vi "Illuminace (SubVI).vi"(5 "R Offset":dbl, 6 "Interval":dbl=1.0, 7 "IR Offset":dbl, 8 "Period (> 3s)":dbl=10.0, 9 "Width":i32, 10 "% Threshold":dbl, 11 "Filtered Signal":dynamicdata(waveform)) -> (0 "waveform out":waveform(dbl), 1 "Imax IR":dbl, 2 "Imin R":dbl, 3 "Imax R":dbl, 4 "Imin IR":dbl)   [LabVIEW 2021]
uses:
  <vilib>/Analysis/baseanly.llb/Mean (DBL).vi
  <vilib>/Waveform/WDTOps.llb/WDT Get Waveform Subset DBL.vi
  <vilib>/Analysis/NI_AAL_SigProc.lvlib
  <vilib>/Analysis/NI_AALBase.lvlib
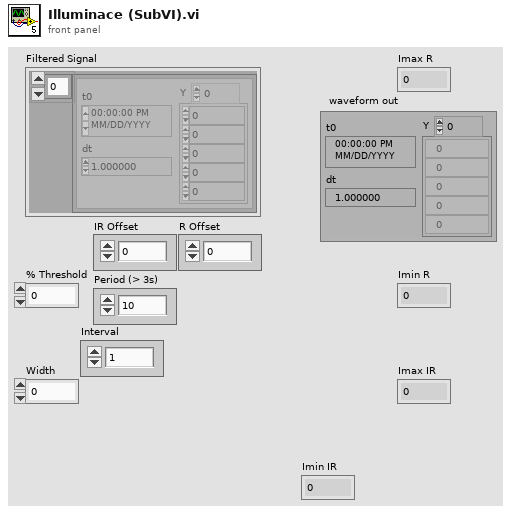
[diagram p1: front panel]
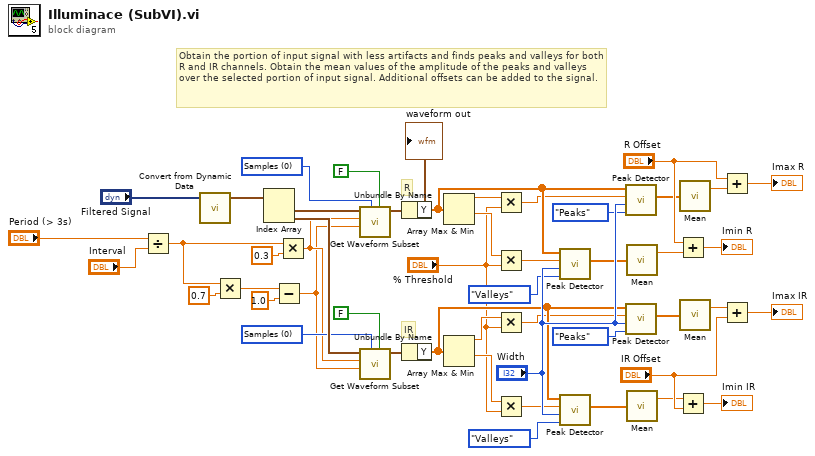
[diagram p0: block diagram]
diagram:
  w12 = u16 0 items=["Samples", "Relative Time"] ("start/duration format")
  w13 = u16 0 items=["Samples", "Relative Time"] ("start/duration format")
  # "Obtain the portion of input signal with less artifacts and finds peaks and valleys for both R and IR channels. Obtain the mean values of the amplitude of the peaks and valleys over the selected portion of input signal. Additional offsets can be added to the signal."
  # "IR"
  # "R"
  n1 = Divide(x="Period (> 3s)", y="Interval") -> (x/y=w3:dbl)
  n2 = call "Convert from Dynamic Data"("Dynamic Data Type"="Filtered Signal") -> ("Array of Waveform"=w33:waveform(dbl)[])  [unwired: 3 in]
  n3 = Multiply(x=w3, y=0.7) -> (x*y=w2:dbl)
  n4 = Index Array(array=w33) -> (element #1=w17:waveform(dbl), element #2=w16:waveform(dbl))  [unwired: 2 in]
  n5 = Subtract(x=w2, y=1.0) -> (x-y=w1:dbl)
  n6 = Multiply(x=w3, y=0.3) -> (x*y=w8:dbl)
  n7 = call-poly <vilib>:"Get Waveform Subset.vi"("open interval? (T)"=FALSE, "start/duration format"=w12, "duration"=w1, "start samples/time"=w8, "waveform in"=w17) -> ("waveform out"=w14:waveform(dbl))  [unwired: 1 in, 3 out]
  "waveform out" <- w14
  n8 = call-poly <vilib>:"Get Waveform Subset.vi"("open interval? (T)"=FALSE, "start/duration format"=w13, "duration"=w1, "start samples/time"=w8, "waveform in"=w16) -> ("waveform out"=w15:waveform(dbl))  [unwired: 1 in, 3 out]
  n9 = Unbundle By Name(w14) -> ("Y"=w28:dbl[])
  n10 = Unbundle By Name(w15) -> ("Y"=w27:dbl[])
  n11 = Array Max & Min(array=w28) -> (max value=w26:dbl, min value=w21:dbl)  [unwired: 2 out]
  n12 = Array Max & Min(array=w27) -> (max value=w25:dbl, min value=w22:dbl)  [unwired: 2 out]
  n13 = Multiply(x=w26, y="% Threshold") -> (x*y=w24:dbl)
  n14 = Multiply(x=w21, y="% Threshold") -> (x*y=w19:dbl)
  n15 = Multiply(x=w25, y="% Threshold") -> (x*y=w23:dbl)
  n16 = Multiply(x=w22, y="% Threshold") -> (x*y=w18:dbl)
  n17 = call <vilib>:"Peak Detector.vi"("peaks/valleys"=enum32{"Peaks", "Valleys"}."Valleys", "width"="Width", "threshold"=w19, "X"=w28) -> ("Amplitudes"=w32:dbl[])  [unwired: 3 in, 4 out]
  n18 = call <vilib>:"Peak Detector.vi"("peaks/valleys"=enum32{"Peaks", "Valleys"}."Valleys", "width"="Width", "threshold"=w18, "X"=w27) -> ("Amplitudes"=w29:dbl[])  [unwired: 3 in, 4 out]
  n19 = call <vilib>:"Peak Detector.vi"("peaks/valleys"=enum32{"Peaks", "Valleys"}."Peaks", "width"="Width", "threshold"=w24, "X"=w28) -> ("Amplitudes"=w31:dbl[])  [unwired: 3 in, 4 out]
  n20 = call <vilib>:"Peak Detector.vi"("peaks/valleys"=enum32{"Peaks", "Valleys"}."Peaks", "width"="Width", "threshold"=w23, "X"=w27) -> ("Amplitudes"=w30:dbl[])  [unwired: 3 in, 4 out]
  n21 = call-poly <vilib>:"Mean.vi"("X"=w32) -> ("mean"=w42:dbl)  [unwired: 1 out]
  n22 = call-poly <vilib>:"Mean.vi"("X"=w29) -> ("mean"=w38:dbl)  [unwired: 1 out]
  n23 = Add(x="R Offset", y=w42) -> (x+y=→"Imin R":dbl)
  n24 = Add(x=w38, y="IR Offset") -> (x+y=→"Imin IR":dbl)
  n25 = call-poly <vilib>:"Mean.vi"("X"=w31) -> ("mean"=w44:dbl)  [unwired: 1 out]
  n26 = call-poly <vilib>:"Mean.vi"("X"=w30) -> ("mean"=w37:dbl)  [unwired: 1 out]
  n27 = Add(x="R Offset", y=w44) -> (x+y=→"Imax R":dbl)
  n28 = Add(x=w37, y="IR Offset") -> (x+y=→"Imax IR":dbl)
